vi "RM-execute-command.vi"(8 "error in (no error)":errorcluster, 10 "command index":u16, 11 "MB_Master_Serial输入":refnum<class "MB_Master_Serial.lvclass">) -> (0 "error out":errorcluster, 3 "MB_Master_Serial输出":refnum<class "MB_Master_Serial.lvclass">)   [LabVIEW 2014]
uses:
  <vilib>/Plasmionique/MB Master/MB_Master_Serial/MB_Master_Serial.lvclass
  <vilib>/Plasmionique/MB Master/MB Master.lvlib
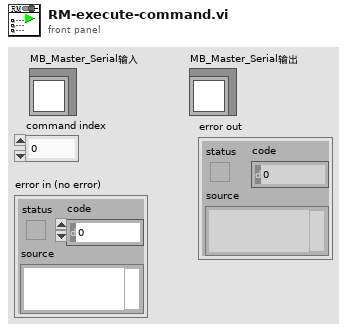
[diagram p1: front panel]
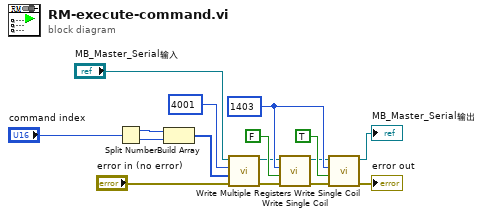
[diagram p0: block diagram]
diagram:
  w9 = u16 1403 ("address")
  n1 = Split Number(x="command index") -> (hi(x)=w12:u8, lo(x)=w11:u8)
  n2 = Build Array(w12, w11) -> (w13:u8[])
  n3 = call <vilib>:"Write Multiple Registers.vi"("error in (no error)"="error in (no error)", "values"=w13, "starting address"=u16 4001, "MB session in"="MB_Master_Serial输入") -> ("error out"=w4:errorcluster, "MB session out"=w3:refnum<class "MB_Master_Serial.lvclass">)  [unwired: 6 in]
  n4 = call <vilib>:"Write Single Coil.vi"("error in (no error)"=w4, "value"=FALSE, "address"=w9, "MB session in"=w3) -> ("error out"=w6:errorcluster, "MB session out"=w7:refnum<class "MB_Master_Serial.lvclass">)  [unwired: 6 in]
  n5 = call <vilib>:"Write Single Coil.vi"("error in (no error)"=w6, "value"=TRUE, "address"=w9, "MB session in"=w7) -> ("error out"=→"error out":errorcluster, "MB session out"=→"MB_Master_Serial输出":refnum<class "MB_Master_Serial.lvclass">)  [unwired: 6 in]
